vi "second_order_system.run.vi"(4 "reset? (F)":bool, 6 "output_limits (100/0)":cluster{"max_limit":dbl, "min_limit":dbl}={"max_limit"=100.0, "min_limit"=0.0}, 7 "transfer_function_parameters":T1={"gain (K)"=1.0, "natural_freq (wn in Hz)"=75.0, "damping_ratio (zeta)"=0.04}, 8 "sampling_time (s)":dbl, 11 "input":dbl format="%#_13g") -> (3 "output":dbl)   [LabVIEW 2015, in "discrete_control_systems.lvlib"]
doc: "Implements a second order transfer function using the provided Gain (K), Natural Frequency (wn), and Damping Ratio (zeta) paramenters and the sampling time. This transfer function can be used directly to simulate the behavior of a plant with second-order response.\n\nThe implemented transfer function has the following equation in the LaPlace domain, where Y(s) is the transfer function output given a U(s) intput:\n\nY(s) K * wn^2\n---- = ----------------------------\nU(s) s^2 + 2*zeta*wn + wn^2 \n\nThe sampling_time input represents how fast will the control loop run and is necessary in order to allow for an accurate implementation of the controller with parameters that can be reused for multiple sampling times.\n\nThe reset? input can be used to reinitialize the internal registers for the controller and start from zero.\n\nThe output will be coerced withing min_limit and max_limit. After resetting the controller, the output will be initialized to the initial output selected. This helps implement bumpless transfers between open loop and closed loop operations."
uses:
  discrete_control_systems.lvlib
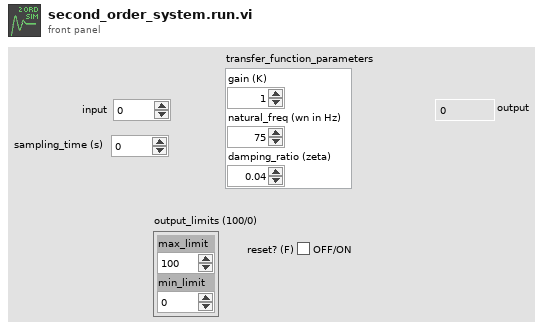
[diagram p1: front panel]
types:
  T1 = cluster{"gain (K)":dbl, "natural_freq (wn in Hz)":dbl, "damping_ratio (zeta)":dbl}
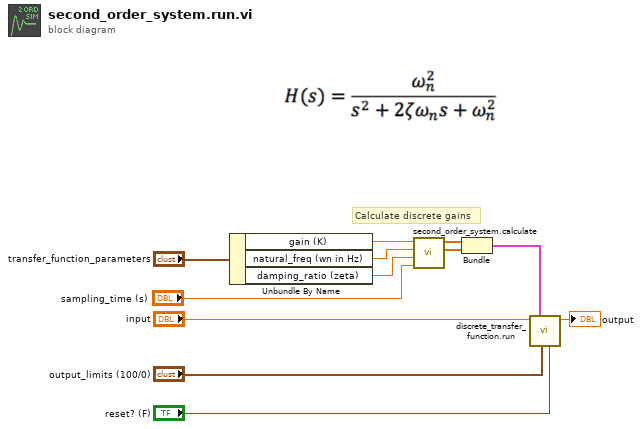
[diagram p0: block diagram]
diagram:
  # "Calculate discrete gains"
  n1 = Unbundle By Name("transfer_function_parameters") -> ("gain (K)"=w11:dbl, "natural_freq (wn in Hz)"=w10:dbl, "damping_ratio (zeta)"=w9:dbl)
  n2 = call "second_order_system.calculate.vi"("sampling_time (s)"="sampling_time (s)", "damping_ratio (zeta)"=w9, "natural_freq (wn in Hz)"=w10, "gain (K)"=w11) -> ("a1...an"=w3:dbl[], "b0...bn"=w4:dbl[])  [unwired: 6 in]
  n3 = Bundle("b0...bn"=w4, "a1...an"=w3) -> (w2:cluster{"b0...bn":dbl[], "a1...an":dbl[]})  [unwired: 1 in]
  n4 = call "discrete_transfer_function.run.vi"("reset? (F)"="reset? (F)", "outut limits (100/0)"="output_limits (100/0)", "discrete_coefficients"=w2, "input"="input") -> ("output"=→"output":dbl)  [unwired: 7 in]
